vi "Test_WriteItem_DeleteItemWrongType_ErrorAndNotRemoved.vi"(8 "error in (no error)":errorcluster, 11 "TestCase in":refnum<class "TestComposedLookupTable.lvclass">) -> (0 "error out":errorcluster, 3 "TestCase out":refnum<class "TestComposedLookupTable.lvclass">)   [LabVIEW 2017, in "TestComposedLookupTable.lvclass"]
uses:
  TestComposedLookupTable.lvclass
  Source/LookupTable/LookupTable.lvclass/LookupTable.ctl
  33395e2c-d572-4611-8838-2d4f290e6471.vi
  7c7ee766-f7d5-4af0-81b0-cb89ba9f3c0f.vi
  1cfbb844-61b9-4cfc-99fd-357fcaac5287.vi
  Source/LookupTable/Read Table Reference.vi
  33395e2c-d572-4611-8838-2d4f290e6471.vi/1e025608-1f2c-4b4e-8d1e-e1b260370443.vi
  1cfbb844-61b9-4cfc-99fd-357fcaac5287.vi/122cce1d-1cb4-4883-8fc8-baadf7b1e525.vi
  Source/LookupTable/LookupTable.lvclass
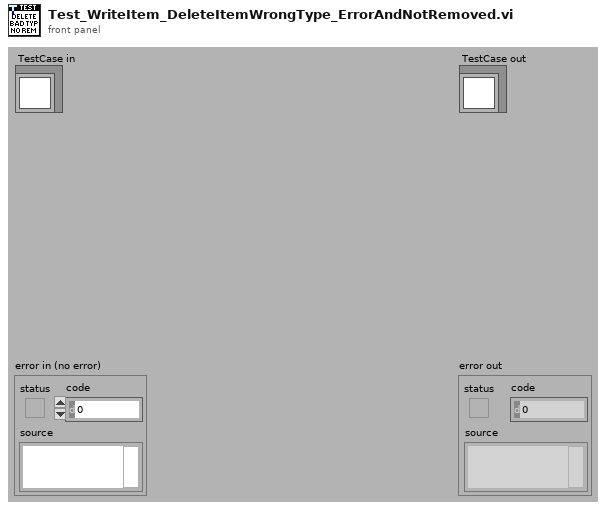
[diagram p1: front panel]
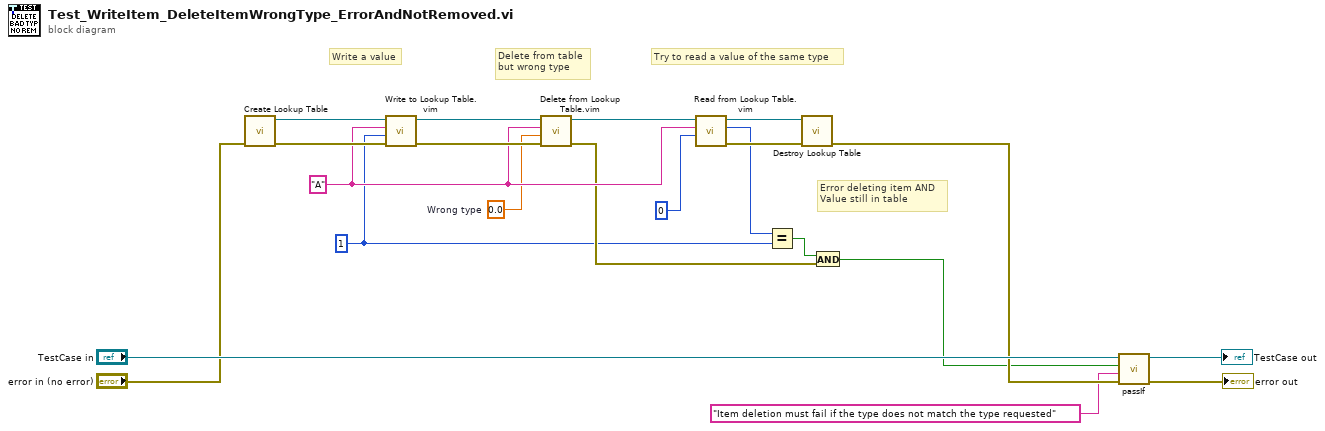
[diagram p0: block diagram]
diagram:
  w7 = 0.0  # Wrong type
  w4 = 1
  w9 = "A" ("Item Name")
  # "Error deleting item AND\nValue still in table"
  # "Delete from table\nbut wrong type"
  # "Try to read a value of the same type"
  # "Write a value"
  n1 = call "Create Lookup Table.vi"("error in (no error)"="error in (no error)") -> ("error out"=w21:errorcluster, "LookupTable Reference"=w16:refnum<data-value>)  [unwired: 9 in]
  n2 = call "Write to Lookup Table.vim"("error in (no error)"=w21, "Item"=w4, "Item Name"=w9, "LookupTable Reference"=w16) -> ("error out"=w20:errorcluster, "LookupTable Reference Out"=w11:refnum<data-value>)  [unwired: 5 in, 1 out]
  n3 = call "Delete from Lookup Table.vim"("error in (no error)"=w20, "Confirm Type"=w7, "Item Name"=w9, "LookupTable Reference"=w11) -> ("error out"=w6:errorcluster, "LookupTable Reference Out"=w10:refnum<data-value>)  [unwired: 5 in, 1 out]
  n4 = call "Read from Lookup Table.vim"("Type"=0, "Item Name"=w9, "LookupTable Reference"=w10) -> ("error out"=w13:errorcluster, "Value"=w5:i32, "LookupTable Reference Out"=w14:refnum<data-value>)  [unwired: 5 in, 1 out]
  n5 = Equal?(x=w5, y=w4) -> (x = y?=w3:bool)
  n6 = call "Destroy Lookup Table.vi"("error in (no error)"=w13, "LookupTable Reference"=w14) -> ("error out"=w12:errorcluster)  [unwired: 9 in]
  n7 = And(x=w3, y=w6) -> (x .and. y?=w2:bool)
  n8 = call-dynamic "passIf.vi"("error in (no error)"=w12, "message (\"\")"="Item deletion must fail if the type does not match the type requested" ("message (\"\")"), "pass"=w2, "TestCase in"="TestCase in") -> ("error out"=→"error out":errorcluster, "TestCase out"=→"TestCase out":refnum<class "TestComposedLookupTable.lvclass">)  [unwired: 6 in]
